vi "replace tag.vi"(8 "error in":errorcluster, 10 "tag to set":refnum<class "tag descriptor.lvclass">, 11 "tag collection in":refnum<class "tag collection.lvclass">) -> (0 "error out":errorcluster, 3 "tag collection out":refnum<class "tag collection.lvclass">)   [LabVIEW 2013, in "tag bus.lvlib" / "tag collection.lvclass"]
uses:
  tag collection.lvclass
  tag/tag descriptor.lvclass
  tag collection.lvclass/tag collection.ctl
  tag/tag descriptor.lvclass/tag descriptor.ctl
  tag bus.lvlib
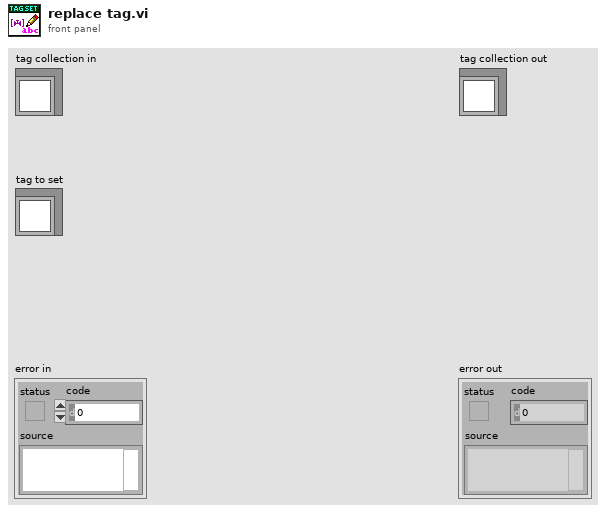
[diagram p1: front panel]
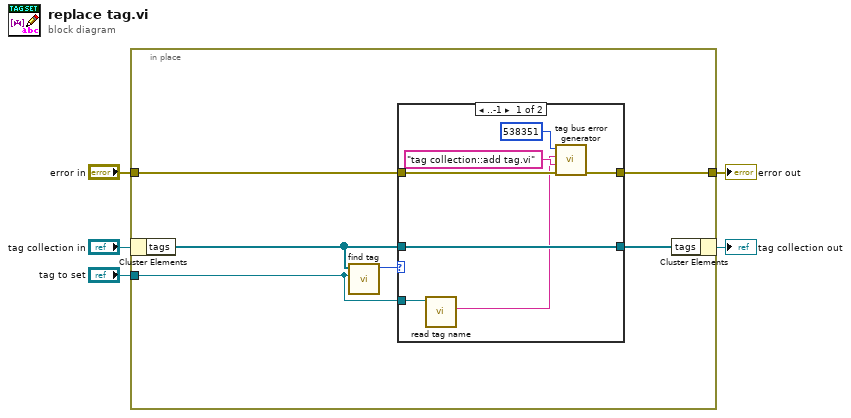
[diagram p0: block diagram]
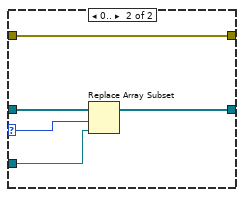
[diagram p2: hidden frame]
diagram:
  n1 = in-place {
    in-place-border: "error in" -> [w10]
    in-place-border: [w11] -> w2
    in-place-border: "tag to set" -> [w7]
    n2 = in-place-cluster #1("tag collection in") -> ("tags"=w8:refnum<class "tag descriptor.lvclass">[])
    n3 = call "find tag.vi"("tag"=w7, "tags in"=w8) -> ("index"=w6:i32)  [unwired: 9 in]
    n4 = case shown="..-1" w6 {
      selector: w6 -> [_ w19]
      tunnel: [w18 w22] -> w9
      tunnel: w8 -> [w18 w23]
      tunnel: [w15 w21] -> w11
      tunnel: w10 -> [w14 w21]
      tunnel: w7 -> [w13 w20]
      frame ..-1 {
        n5 = call "read tag name.vi"("system tag in"=w13) -> ("name"=w12:string)  [unwired: 8 in, 2 out]
        n6 = call "tag bus error generator.vi"("error in"=w14, "source"="tag collection::add tag.vi", "append error message"=w12, "error code (0)"=538351) -> ("error out"=w15:errorcluster)  [unwired: 5 in]
      }
      frame 0.. {
        n7 = Replace Array Subset(array=w23, new element=w20, index=w19) -> (w22:refnum<class "tag descriptor.lvclass">[])
      }
    }
    n8 = in-place-cluster #1("tags"=w9) -> (→"tag collection out":refnum<class "tag collection.lvclass">)
  }
  "error out" <- w2
